vi "Do Recombination.vi"(8 "error in":errorcluster, 9 "IChromosome Parent B in":refnum<class "IChromosome.lvclass">, 10 "IChromosome Parent A in":refnum<class "IChromosome.lvclass">, 11 "Recombinator in":refnum<class "Recombinator.lvclass">) -> (0 "error out":errorcluster, 1 "IChromosome Child B out":refnum<class "IChromosome.lvclass">, 2 "IChromosome Child A out":refnum<class "IChromosome.lvclass">, 3 "Recombinator out":refnum<class "Recombinator.lvclass">)   [LabVIEW 2016, in "Recombinator.lvclass"]
uses:
  Recombinator.lvclass
  IChromosome/IChromosome.lvclass
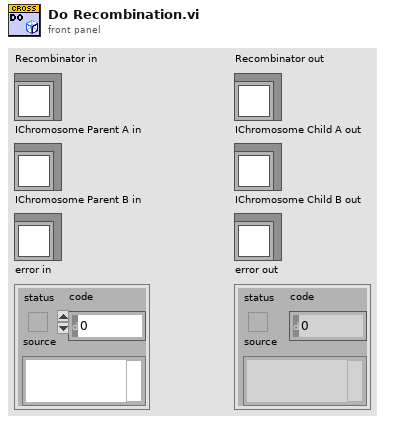
[diagram p1: front panel]
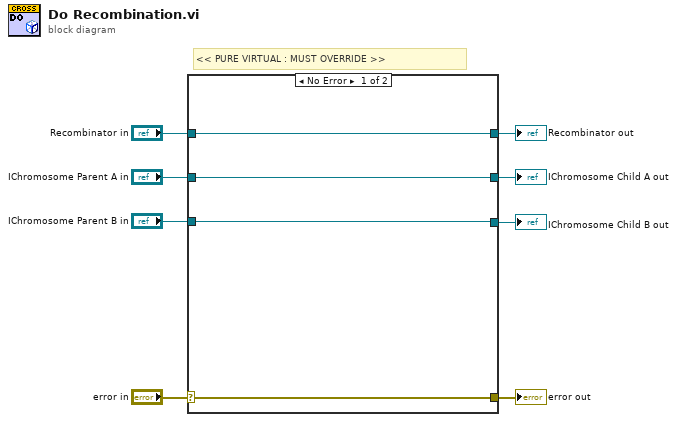
[diagram p0: block diagram]
diagram:
  # "<< PURE VIRTUAL : MUST OVERRIDE >>"
  n1 = case shown="No Error" "error in" {
    selector: "error in" -> [w11 w16]
    tunnel: [w11 w16] -> w7
    tunnel: [w12 w15] -> w5
    tunnel: "Recombinator in" -> [w12 w15]
    tunnel: "IChromosome Parent A in" -> [w10 w14]
    tunnel: "IChromosome Parent B in" -> [w9 w13]
    tunnel: [w10 w14] -> w2
    tunnel: [w9 w13] -> w1
    frame No Error {
    }
    frame Error {
    }
  }
  "error out" <- w7
  "Recombinator out" <- w5
  "IChromosome Child B out" <- w1
  "IChromosome Child A out" <- w2
